vi "Read Setting.vi"(8 "error in":errorcluster, 11 "PRM in":refnum<class "PRM.lvclass">) -> (0 "error out":errorcluster, 2 "Setting":dbl, 3 "PRM out":refnum<class "PRM.lvclass">)   [LabVIEW 2019, in "PRM.lvlib" / "PRM.lvclass"]
uses:
  Library/PRM.lvclass
  Library/PRM.lvclass/PRM.ctl
  Read Active Channel.vi
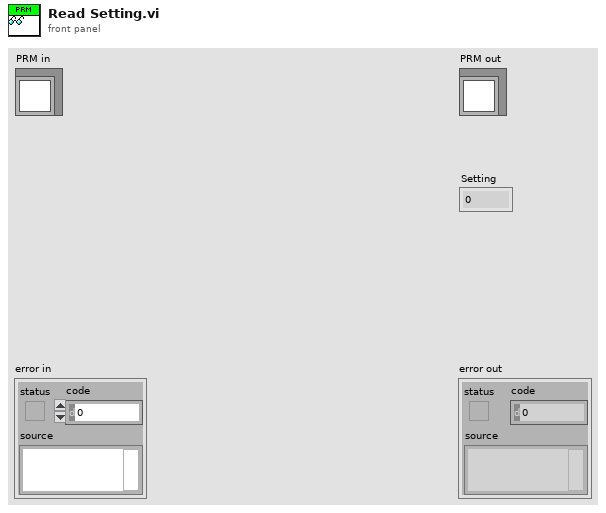
[diagram p1: front panel]
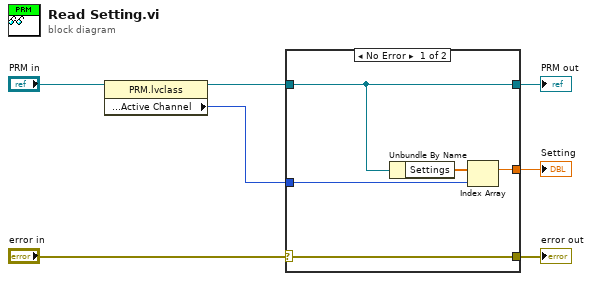
[diagram p0: block diagram]
diagram:
  n1 = property class="PRM.lvclass"(reference="PRM in") -> (reference out=w2:refnum<class "PRM.lvclass">, "Accessors:Settings:Active Channel"=w1:u32)  [unwired: 1 in, 1 out]
  n2 = case shown="No Error" "error in" {
    selector: "error in" -> [w12 w13]
    tunnel: [w12 w13] -> w6
    tunnel: [w11 w14] -> w4
    tunnel: w2 -> [w11 w14]
    tunnel: [w9 _] -> w3
    tunnel: w1 -> [w8 _]
    frame No Error {
      n3 = Unbundle By Name(w11) -> ("Settings"=w10:dbl[])
      n4 = Index Array(array=w10, index=w8) -> (element=w9:dbl)
    }
    frame Error {
    }
  }
  "error out" <- w6
  "PRM out" <- w4
  "Setting" <- w3
